vi "USB2XXX_K_Test.vi"() -> ()   [LabVIEW 2010]
panel:
  in  "ResponseTimeOutMs":i32=1000
  in  "InterByteTimeMs":u8=5
  in  "pResponse":T1
  out "pResponse out":T1
  in  "pRequest":T1
  out "pRequest out":T1
  out "function return":i32
  out "KB1 Out":u8 format="%x"
  out "KB2 Out":u8 format="%x"
  in  "KB2":u8 format="%x"
  in  "KB1":u8 format="%x"
  in  "TgtAddr":u8=51 format="%x"
  in  "BaudRate":i32=10400
  in  "Channel":u8
  in  "Device Index":i32(ring) items=["0", "1", "2", "3", "4", "5"]
  # "波特率一定要设置，否则程序可能出错"
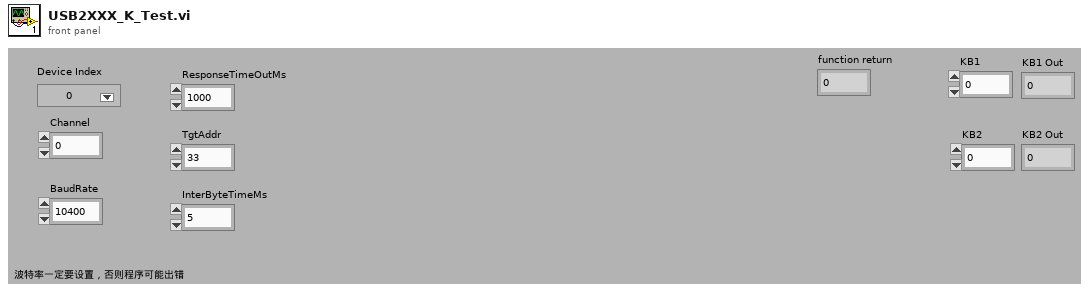
[diagram p1: front panel]
types:
  T1 = cluster{"Fmt":u8, "TgtAddr":u8, "SrcAddr":u8, "Len":u8, "SId":u8, "Data[0]":u8, "Data[1]":u8, "Data[2]":u8, "Data[3]":u8, "Data[4]":u8, "Data[5]":u8, "Data[6]":u8, "Data[7]":u8, "Data[8]":u8, "Data[9]":u8, "Data[10]":u8, "Data[11]":u8, "Data[12]":u8, "Data[13]":u8, "Data[14]":u8, "Data[15]":u8, "Data[16]":u8, "Data[17]":u8, "Data[18]":u8, "Data[19]":u8, "Data[20]":u8, "Data[21]":u8, "Data[22]":u8, "Data[23]":u8, "Data[24]":u8, "Data[25]":u8, "Data[26]":u8, "Data[27]":u8, "Data[28]":u8, "Data[29]":u8, "Data[30]":u8, "Data[31]":u8, "Data[32]":u8, "Data[33]":u8, "Data[34]":u8, "Data[35]":u8, "Data[36]":u8, "Data[37]":u8, "Data[38]":u8, "Data[39]":u8, "Data[40]":u8, "Data[41]":u8, "Data[42]":u8, "Data[43]":u8, "Data[44]":u8, "Data[45]":u8, "Data[46]":u8, "Data[47]":u8, "Data[48]":u8, "Data[49]":u8, "Data[50]":u8, "Data[51]":u8, "Data[52]":u8, "Data[53]":u8, "Data[54]":u8, "Data[55]":u8, "Data[56]":u8, "Data[57]":u8, "Data[58]":u8, "Data[59]":u8, "Data[60]":u8, "Data[61]":u8, "Data[62]":u8, "Data[63]":u8, "Data[64]":u8, "Data[65]":u8, "Data[66]":u8, "Data[67]":u8, "Data[68]":u8, "Data[69]":u8, "Data[70]":u8, "Data[71]":u8, "Data[72]":u8, "Data[73]":u8, "Data[74]":u8, "Data[75]":u8, "Data[76]":u8, "Data[77]":u8, "Data[78]":u8, "Data[79]":u8, "Data[80]":u8, "Data[81]":u8, "Data[82]":u8, "Data[83]":u8, "Data[84]":u8, "Data[85]":u8, "Data[86]":u8, "Data[87]":u8, "Data[88]":u8, "Data[89]":u8, "Data[90]":u8, "Data[91]":u8, "Data[92]":u8, "Data[93]":u8, "Data[94]":u8, "Data[95]":u8, "Data[96]":u8, "Data[97]":u8, "Data[98]":u8, "Data[99]":u8, "Data[100]":u8, "Data[101]":u8, "Data[102]":u8, "Data[103]":u8, "Data[104]":u8, "Data[105]":u8, "Data[106]":u8, "Data[107]":u8, "Data[108]":u8, "Data[109]":u8, "Data[110]":u8, "Data[111]":u8, "Data[112]":u8, "Data[113]":u8, "Data[114]":u8, "Data[115]":u8, "Data[116]":u8, "Data[117]":u8, "Data[118]":u8, "Data[119]":u8, "Data[120]":u8, "Data[121]":u8, "Data[122]":u8, "Data[123]":u8, "Data[124]":u8, "Data[125]":u8, "Data[126]":u8, "Data[127]":u8, "Data[128]":u8, "Data[129]":u8, "Data[130]":u8, "Data[131]":u8, "Data[132]":u8, "Data[133]":u8, "Data[134]":u8, "Data[135]":u8, "Data[136]":u8, "Data[137]":u8, "Data[138]":u8, "Data[139]":u8, "Data[140]":u8, "Data[141]":u8, "Data[142]":u8, "Data[143]":u8, "Data[144]":u8, "Data[145]":u8, "Data[146]":u8, "Data[147]":u8, "Data[148]":u8, "Data[149]":u8, "Data[150]":u8, "Data[151]":u8, "Data[152]":u8, "Data[153]":u8, "Data[154]":u8, "Data[155]":u8, "Data[156]":u8, "Data[157]":u8, "Data[158]":u8, "Data[159]":u8, "Data[160]":u8, "Data[161]":u8, "Data[162]":u8, "Data[163]":u8, "Data[164]":u8, "Data[165]":u8, "Data[166]":u8, "Data[167]":u8, "Data[168]":u8, "Data[169]":u8, "Data[170]":u8, "Data[171]":u8, "Data[172]":u8, "Data[173]":u8, "Data[174]":u8, "Data[175]":u8, "Data[176]":u8, "Data[177]":u8, "Data[178]":u8, "Data[179]":u8, "Data[180]":u8, "Data[181]":u8, "Data[182]":u8, "Data[183]":u8, "Data[184]":u8, "Data[185]":u8, "Data[186]":u8, "Data[187]":u8, "Data[188]":u8, "Data[189]":u8, "Data[190]":u8, "Data[191]":u8, "Data[192]":u8, "Data[193]":u8, "Data[194]":u8, "Data[195]":u8, "Data[196]":u8, "Data[197]":u8, "Data[198]":u8, "Data[199]":u8, "Data[200]":u8, "Data[201]":u8, "Data[202]":u8, "Data[203]":u8, "Data[204]":u8, "Data[205]":u8, "Data[206]":u8, "Data[207]":u8, "Data[208]":u8, "Data[209]":u8, "Data[210]":u8, "Data[211]":u8, "Data[212]":u8, "Data[213]":u8, "Data[214]":u8, "Data[215]":u8, "Data[216]":u8, "Data[217]":u8, "Data[218]":u8, "Data[219]":u8, "Data[220]":u8, "Data[221]":u8, "Data[222]":u8, "Data[223]":u8, "Data[224]":u8, "Data[225]":u8, "Data[226]":u8, "Data[227]":u8, "Data[228]":u8, "Data[229]":u8, "Data[230]":u8, "Data[231]":u8, "Data[232]":u8, "Data[233]":u8, "Data[234]":u8, "Data[235]":u8, "Data[236]":u8, "Data[237]":u8, "Data[238]":u8, "Data[239]":u8, "Data[240]":u8, "Data[241]":u8, "Data[242]":u8, "Data[243]":u8, "Data[244]":u8, "Data[245]":u8, "Data[246]":u8, "Data[247]":u8, "Data[248]":u8, "Data[249]":u8, "Data[250]":u8, "Data[251]":u8, "Data[252]":u8, "Data[253]":u8, "CS":u8}
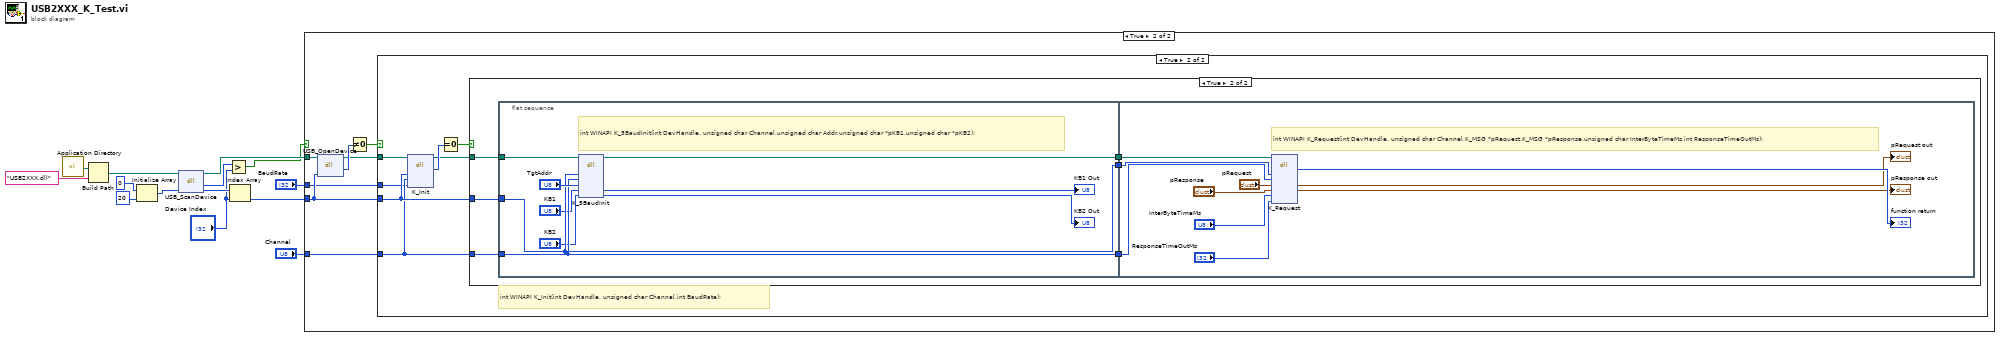
[diagram p0: block diagram]
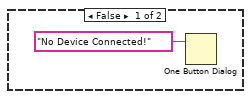
[diagram p2: hidden frame]
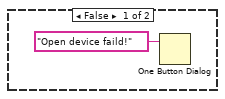
[diagram p3: hidden frame]
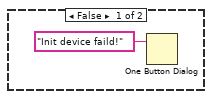
[diagram p4: hidden frame]
diagram:
  n1 = call <vilib>:"Application Directory.vi"() -> ("Application Directory"=w5:path)
  n2 = Build Path(base path=w5, name or relative path="USB2XXX.dll") -> (appended path=w4:path)
  n3 = Initialize Array(0, 20 ("dimension size")) -> (w12:i32[])
  n4 = dll-call lib="E:/OtherWork/STM32/USB2XXX_Example/examples/Labview/PublicFiles/USB2XXX.dll" fn="USB_ScanDevice"(path in=w4, "pDevNum"=w12) -> (path out=w10:path, "return type"=w2:i32, "pDevNum"=w11:i32[])  [unwired: 2 in, 1 out]
  n5 = Greater?(x=w2, y="Device Index") -> (0:w3:bool)
  n6 = Index Array(array=w11, index="Device Index") -> (element=w9:i32)
  n7 = case shown="True" w3 {
    tunnel: w10 -> [_ w22]
    tunnel: w9 -> [_ w18]
    tunnel: "Channel" -> [_ w17]
    tunnel: "BaudRate" -> [_ w16]
    frame False {
      n8 = One Button Dialog(message="No Device Connected!") -> ()  [unwired: 1 in, 1 out]
    }
    frame True {
      n9 = dll-call lib="E:/OtherWork/STM32/USB2XXX_Example/examples/Labview/PublicFiles/USB2XXX.dll" fn="USB_OpenDevice"(path in=w22, "DevIndex"=w18) -> (path out=w19:path, "return type"=w21:u8)  [unwired: 3 in, 1 out]
      n10 = Not Equal To 0?(x=w21) -> (x != 0?=w20:bool)
      n11 = case shown="True" w20 {
        tunnel: w19 -> [_ w29]
        tunnel: w18 -> [_ w28]
        tunnel: w17 -> [_ w27]
        tunnel: w16 -> [_ w24]
        frame False {
          n12 = One Button Dialog(message="Open device faild!") -> ()  [unwired: 1 in, 1 out]
        }
        frame True {
          # "int WINAPI K_Init(int DevHandle, unsigned char Channel,int BaudRate);"
          n13 = dll-call lib="E:/OtherWork/STM32/USB2XXX_Example/examples/Labview/PublicFiles/USB2XXX.*" fn="K_Init"(path in=w29, "DevHandle"=w28, "Channel"=w27, "BaudRate"=w24) -> (path out=w25:path, "return type"=w26:i32)  [unwired: 5 in, 1 out]
          n14 = Equal To 0?(x=w26) -> (x = 0?=w30:bool)
          n15 = case shown="True" w30 {
            tunnel: w25 -> [_ w37]
            tunnel: w28 -> [_ w36]
            tunnel: w27 -> [_ w35]
            frame False {
              n16 = One Button Dialog(message="Init device faild!") -> ()  [unwired: 1 in, 1 out]
            }
            frame True {
              n17 = flat-sequence {
                tunnel: w37 -> [w45]
                tunnel: w36 -> [w44]
                tunnel: w35 -> [w43]
                tunnel: [w44] -> w34
                tunnel: [w43] -> w33
                tunnel: [w38] -> w32
                tunnel: w34 -> [w48]
                tunnel: w33 -> [w47]
                tunnel: w32 -> [w49]
                frame #0 {
                  # "int WINAPI K_5BaudInit(int DevHandle, unsigned char Channel,unsigned char Addr,unsigned char *pKB1,unsigned char *pKB2);"
                  n18 = dll-call lib="E:/Projects/USB2XXX_Example/sdk/api/Labview/USB2XXX.*" fn="K_5BaudInit"(path in=w45, "DevHandle"=w44, "Channel"=w43, "Addr"="TgtAddr", "pKB1"="KB1", "pKB2"="KB2") -> (path out=w38:path, "pKB1"=→"KB1 Out":u8, "pKB2"=→"KB2 Out":u8)  [unwired: 6 in, 1 out]
                }
                frame #1 {
                  # "int WINAPI K_Request(int DevHandle, unsigned char Channel,K_MSG *pRequest,K_MSG *pResponse,unsigned char InterByteTimeMs,int ResponseTimeOutMs);"
                  n19 = dll-call lib="E:/Projects/USB2XXX_Example/sdk/api/Labview/USB2XXX.*" fn="K_Request"(path in=w49, "DevHandle"=w48, "Channel"=w47, "pRequest"="pRequest", "pResponse"="pResponse", "InterByteTimeMs"="InterByteTimeMs", "ResponseTimeOutMs"="ResponseTimeOutMs") -> ("return type"=→"function return":i32, "pRequest"=→"pRequest out":T1, "pResponse"=→"pResponse out":T1)  [unwired: 6 in, 2 out]
                }
              }
            }
          }
        }
      }
    }
  }
